vi "dsymv - Symmetric Matrix-Vector Product (DBL).vi"(4 "beta":dbl=1.0, 6 "alpha":dbl=1.0, 8 "matrix A type":T1=3 items=["Lower Triangular"=2, "Upper Triangular"=3], 9 "y":dbl[](array[numeric]), 10 "x":dbl[](array[numeric]), 11 "A":T2) -> (0 "error":i32, 3 "dsymv":dbl[](array[numeric]))   [LabVIEW 2017, in "NI_AALBLAS.lvlib"]
doc: "Calculates the product of a symmetric matrix and a vector."
uses:
  NI_AALBLAS.lvlib
  RealMatrix.ctl
  LV_UpLo.ctl
  Order.ctl
  Fucntion.ctl
  BLAS2 Utility(DBL).vi
  NI_Matrix.lvlib
panel:
  # "dsymv=alpha*A*x+beta*y"
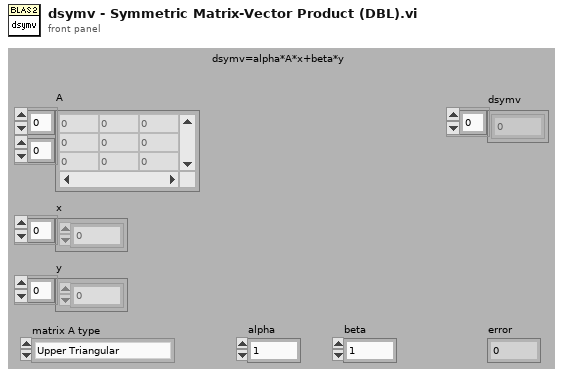
[diagram p1: front panel]
types:
  T1 = typedef "NI_AALBLAS.lvlib/LV_UpLo.ctl" = i32
  T2 = typedef "NI_Matrix.lvlib/RealMatrix.ctl" = dbl[][]
  T3 = typedef "NI_AALBLAS.lvlib/Fucntion.ctl" = u16
  T4 = typedef "NI_AALBLAS.lvlib/Order.ctl" = i32
  T5 = typedef "NI_AALBLAS.lvlib/UpLo.ctl" = i32
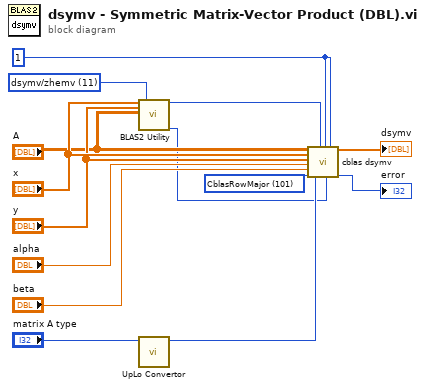
[diagram p0: block diagram]
diagram:
  w1 = 1
  w2 = T3 11 items=["ddot/zdotu/zdotc", "daxpy/zaxpy", "dnrm2/dznrm2", "dasum/dzasum", "dcopy/zcopy", "dswap/zswap", "drotm", "drot/zdrot", "idamax/izamax", "idamin/izamin", "dgemv/zgemv", "dsymv/zhemv", "dtrmv/ztrmv", "dsyr/zher", "dsyr2/zher2", "dger/zgeru/zgerc", "dtrsv/ztrsv", "dgemm/zgemm", "dsymm/zsymm/zhemm", "dtrmm/ztrmm", "dsyrk/zsyrk/zherk", "dsyr2k/zsyr2k/zher2k", "dtrsm/ztrsm"] ("function")
  w4 = T4 101 items=["CblasRowMajor"=101, "CblasColMajor"=102] ("order")
  n1 = call-poly "BLAS2 Utility.vi"("x"="x", "y"="y", "A"="A", "function"=w2) -> ("lda"=w5:i32, "n"=w3:i32)  [unwired: 1 in, 13 out]
  n2 = call "UpLo Convertor.vi"("triangle matrix type"="matrix A type") -> ("uplo"=w11:T5)  [unwired: 10 out]
  n3 = call "cblas dsymv.vi"("A"="A", "x"="x", "y"="y", "alpha"="alpha", "beta"="beta", "order"=w4, "uplo"=w11, "lda"=w5, "incx"=w1, "n"=w3, "incy"=w1) -> ("dsymv"=→"dsymv":dbl[], "error"=→"error":i32)  [unwired: 7 out]
